vi "MT Generate CPM System Parameters (M).vi"(0 "samples per symbol (16)":i32=16, 5 "M-CPM (2)":i32=2, 7 "modulation index, h(i)":cluster{"numerator":i32, "denominator":i32}[](array[cluster]), 9 "symbol rate":dbl=1.0, 11 "error in (no error)":errorcluster) -> (6 "CPM system parameters":T1, 8 "bits per symbol":i32, 15 "error out":errorcluster)   [LabVIEW 2020, in "niDMT.lvlib"]
doc: "This polymorphic instance accepts an M-ary value that specifies a predefined symbol map with the number of distinct symbol map values to use as symbols."
uses:
  <vilib>/addons/Modulation/niDMT.lvlib
  <vilib>/addons/Modulation/Digital/Support/Controls/CPM System Parameters.ctl
  <vilib>/Analysis/1siggen.llb/Ramp Pattern by Samples.vi
  <vilib>/addons/Modulation/niAMT.lvlib
  <vilib>/Analysis/NI_AALBase.lvlib
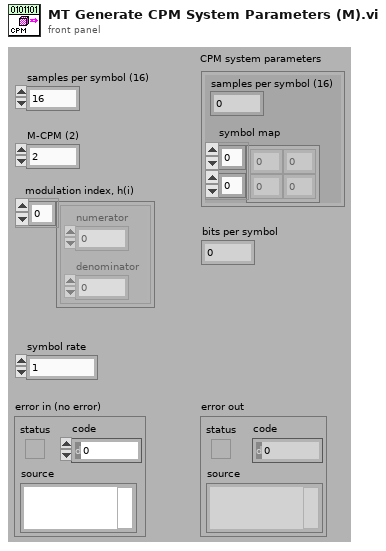
[diagram p1: front panel]
types:
  T1 = typedef "niDMT.lvlib/CPM System Parameters.ctl" = cluster{"samples per symbol (16)":i32, "symbol map":dbl[][]}
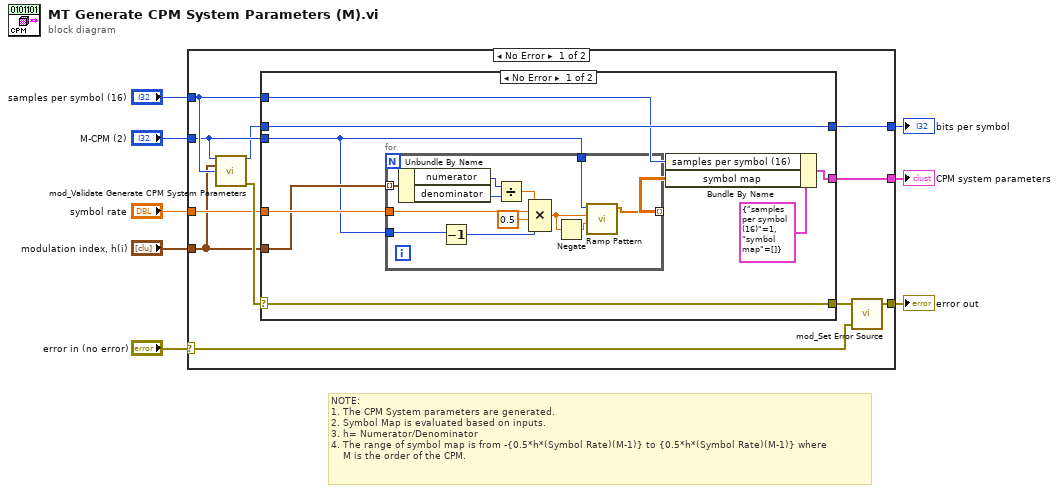
[diagram p0: block diagram]
diagram:
  # "NOTE: \n1. The CPM System parameters are generated. \n2. Symbol Map is evaluated based on inputs. \n3. h= Numerator/Denominator\n4. The range of symbol map is from -{0.5*h*(Symbol Rate)(M-1)} to {0.5*h*(Symbol Rate)(M-1)} where \n    M is the order of the CPM."
  n1 = case shown="No Error" "error in (no error)" {
    selector: "error in (no error)" -> [w10 w42]
    tunnel: "samples per symbol (16)" -> [w16 _]
    tunnel: "M-CPM (2)" -> [w15 _]
    tunnel: [w11 _] -> w6
    tunnel: [w19 _] -> w5
    tunnel: [w18 w42] -> w3
    tunnel: "modulation index, h(i)" -> [w9 _]
    tunnel: "symbol rate" -> [w12 _]
    frame No Error {
      n2 = call <vilib>:"mod_Validate Generate CPM System Parameters.vi"("M-CPM"=w15, "modulation index, h(i)"=w9, "samples per symbol"=w16) -> ("bits per symbol"=w13:i32, "error out"=w14:errorcluster)  [unwired: 11 out]
      n3 = case shown="No Error" w14 {
        selector: w14 -> [w27 w41]
        tunnel: w16 -> [w25 _]
        tunnel: w15 -> [w22 _]
        tunnel: [w28 _] -> w19
        tunnel: [w27 w41] -> w17
        tunnel: w13 -> [w28 _]
        tunnel: w9 -> [w24 _]
        tunnel: w12 -> [w26 _]
        tunnel: [w23 _] -> w11
        frame No Error {
          n4 = for {
            tunnel: w24 -> [w40] mode=indexing
            tunnel: w26 -> [w29]
            tunnel: w22 -> [w33]
            tunnel: [w32] -> w20 mode=indexing
            tunnel: w22 -> [w30]
            n5 = Unbundle By Name(w40) -> ("numerator"=w38:i32, "denominator"=w37:i32)
            n6 = Decrement(x=w30) -> (x-1=w31:i32)
            n7 = Divide(x=w38, y=w37) -> (x/y=w36:dbl)
            n8 = Compound Arithmetic op=MULTIPLY(w36, w29, 0.5 ("value"), w31) -> (w34:dbl)
            n9 = Negate(x=w34) -> (-x=w39:dbl)
            n10 = call-poly <vilib>:"Ramp Pattern.vi"("start"=w39, "end"=w34, "samples"=w33) -> ("Ramp Pattern"=w32:dbl[])  [unwired: 7 in, 1 out]
          }
          n11 = Bundle By Name(cluster=T1 {"samples per symbol (16)"=1, "symbol map"=[]} ("CPM system parameters"), "samples per symbol (16)"=w25, "symbol map"=w20) -> (w23:T1)
        }
        frame Error {
        }
      }
      n12 = call <vilib>:"mod_Set Error Source.vi"("initial error in (no error)"=w10, "final error in (no error)"=w17) -> ("error out"=w18:errorcluster)  [unwired: 3 out]
    }
    frame Error {
    }
  }
  "CPM system parameters" <- w6
  "bits per symbol" <- w5
  "error out" <- w3
